vi "Start Stop Handles Hierarchy to Channels Array.vi"(8 "error in":errorcluster, 11 "1553 start stop handles":T1[](array[typedef]) {"start stop handles"."stop handle" format="%.0x"; "start stop handles"."start handle" format="%.0x"}) -> (0 "error out":errorcluster, 3 "start stop channels":T4[](array[typedef]) format="%.0x")   [LabVIEW 2020, in "Ballard MIL-STD-1553 Engine.lvlib" / "Implementation.lvlib" / "Address Based Execution Unit.lvclass"]
uses:
  Address Based Execution Unit/Address Based Execution Unit.lvclass
  <vilib>/NI VeriStand/Custom Device API/Custom Device Item Ref.ctl
  <vilib>/NI VeriStand/Custom Device API/Custom Device API.lvlib
  Shared/Address.ctl
  Start Stop Channel Handles.ctl
  1553 Start Stop Channel Handles.ctl
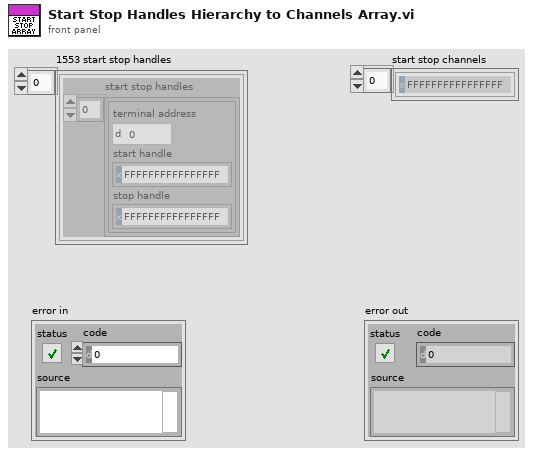
[diagram p1: front panel]
types:
  T1 = typedef "Ballard MIL-STD-1553 Engine.lvlib/Implementation.lvlib/Address Based Execution Unit.lvclass/1553 Start Stop Channel Handles.ctl" = cluster{"start stop handles":T2[]}
  T2 = typedef "Ballard MIL-STD-1553 Engine.lvlib/Implementation.lvlib/Address Based Execution Unit.lvclass/Start Stop Channel Handles.ctl" = cluster{"terminal address":T3, "start handle":T4, "stop handle":T4}
  T3 = typedef "Address.ctl" = u16
  T4 = typedef "Custom Device API.lvlib/Custom Device Item Ref.ctl" = u64
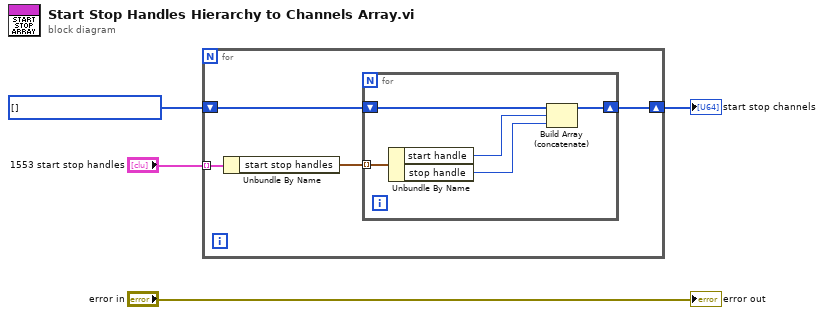
[diagram p0: block diagram]
diagram:
  n1 = for {
    shift-right: [w7] -> w4
    shift-left: T4[] [] ("Incoming Channels") -> [w8]
    tunnel: "1553 start stop handles" -> [w6] mode=indexing
    n2 = Unbundle By Name(w6) -> ("start stop handles"=w5:T2[])
    n3 = for {
      shift-right: [w12] -> w7
      shift-left: w8 -> [w13]
      tunnel: w5 -> [w11] mode=indexing
      n4 = Unbundle By Name(w11) -> ("start handle"=w10:T4, "stop handle"=w9:T4)
      n5 = Build Array (concatenate)(w13, w10, w9) -> (w12:T4[])
    }
  }
  "start stop channels" <- w4
  "error out" <- "error in"
